vi "SeparateNames.vi"(11 "CompleteName":string) -> (3 "SeparateWords":string[](array[string]))   [LabVIEW 2014]
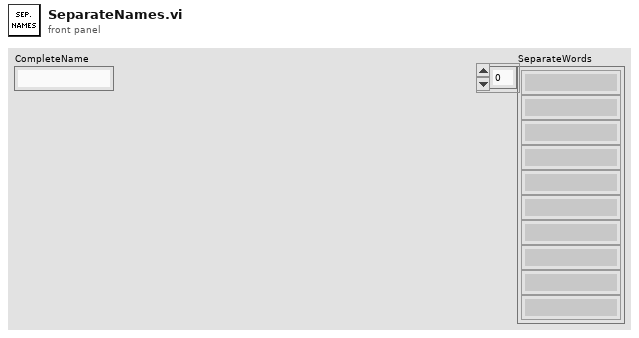
[diagram p1: front panel]
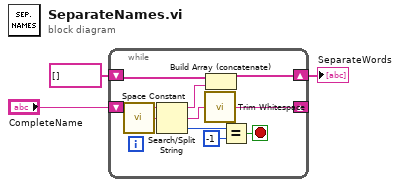
[diagram p0: block diagram]
diagram:
  n1 = while {
    shift-right: [w12] -> w1
    shift-left: string[] [] -> [w13]
    shift-right: [w7] -> _
    shift-left: "CompleteName" -> [w10]
    stop <- w4 stop-if-true
    n2 = call <vilib>:"Space Constant.vi"() -> ("String"=w11:string)
    n3 = Search/Split String(string=w10, search string/char (-)=w11) -> (substring before match=w9:string, match + rest of string=w8:string, offset of match=w6:i32)  [unwired: 1 in]
    n4 = call <vilib>:"Trim Whitespace.vi"("string"=w8) -> ("trimmed string"=w7:string)  [unwired: 1 in]
    n5 = Build Array (concatenate)(w13, w9) -> (w12:string[])
    n6 = Equal?(x=w6, y=-1) -> (x = y?=w4:bool)
  }
  "SeparateWords" <- w1
